vi "Converting the data coming from switches as a boolean to deciamal numbers.vi"() -> ()   [LabVIEW 2024]
panel:
  out "Numeric":dbl
  in  "Boolean 3":bool
  in  "Boolean 2":bool
  in  "Boolean":bool
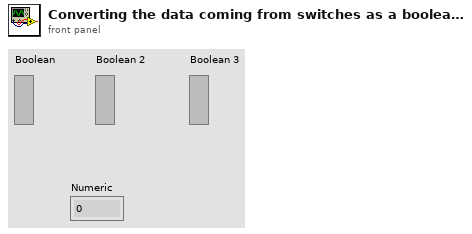
[diagram p1: front panel]
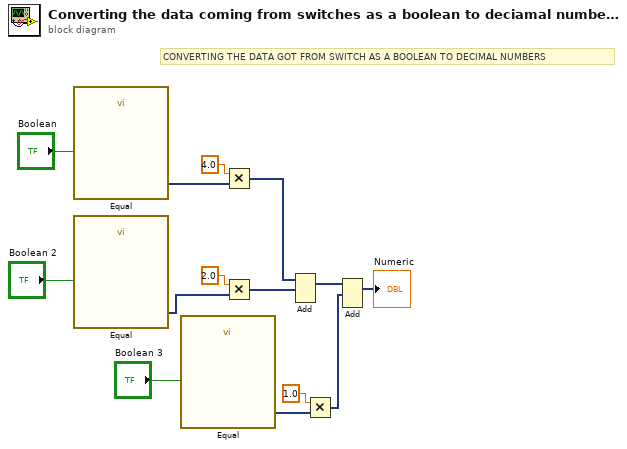
[diagram p0: block diagram]
diagram:
  # "CONVERTING THE DATA GOT FROM SWITCH AS A BOOLEAN TO DECIMAL NUMBERS"
  n1 = call "Equal"("Operand 1"="Boolean") -> ("Result"=w8:dynamicdata)  [unwired: 9 in, 1 out]
  n2 = call "Equal"("Operand 1"="Boolean 2") -> ("Result"=w7:dynamicdata)  [unwired: 9 in, 1 out]
  n3 = call "Equal"("Operand 1"="Boolean 3") -> ("Result"=w6:dynamicdata)  [unwired: 9 in, 1 out]
  n4 = Multiply(x=4.0, y=w8) -> (x*y=w4:dynamicdata)
  n5 = Multiply(x=2.0, y=w7) -> (x*y=w5:dynamicdata)
  n6 = Add(1:w5, 2:w4) -> (0:w2:dynamicdata)  [unwired: 1 in, 1 out]
  n7 = Multiply(x=1.0, y=w6) -> (x*y=w3:dynamicdata)
  n8 = Add(1:w3, 2:w2) -> (0:→"Numeric":dynamicdata)  [unwired: 1 in, 1 out]
